vi "create_current_variables_table.vi"(7 "Step Sizes Array":dbl[](array[numeric]), 8 "error in (no error)":errorcluster, 9 "variable values":dbl[](array[numeric]), 10 "variable indices":i32[](array[numeric]), 11 "Variable Names Array":string[](array[string])) -> (0 "error out":errorcluster, 3 "Variables (Indicator)":string[][](array[string]))   [LabVIEW 2011]
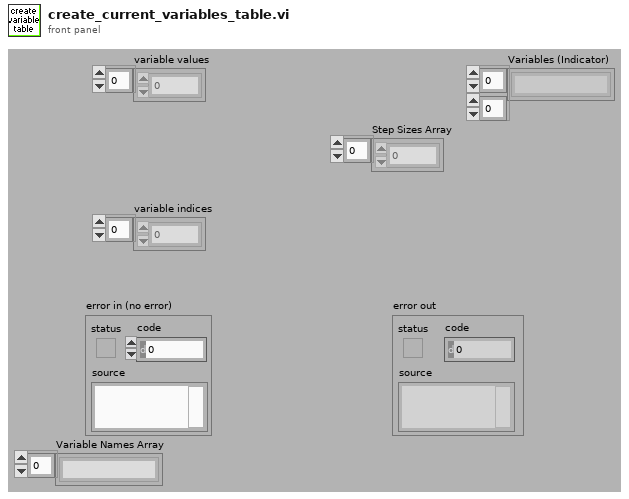
[diagram p1: front panel]
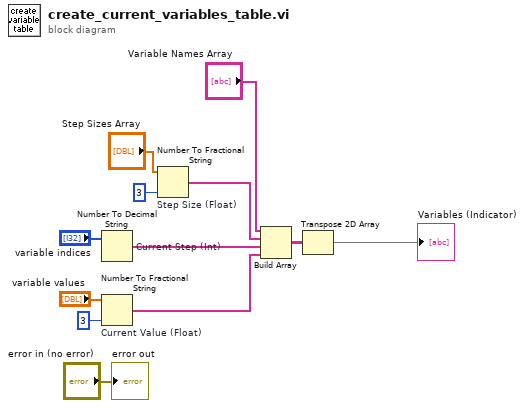
[diagram p0: block diagram]
diagram:
  n1 = Number To Decimal String "Current Step (Int)"(number="variable indices") -> (decimal integer string=w3:string[])  [unwired: 1 in]
  n2 = Number To Fractional String "Current Value (Float)"(number="variable values", precision (6)=i16 3) -> (F-format string=w2:string[])  [unwired: 2 in]
  n3 = Number To Fractional String "Step Size (Float)"(number="Step Sizes Array", precision (6)=i16 3) -> (F-format string=w4:string[])  [unwired: 2 in]
  n4 = Build Array("Variable Names Array", w4, w3, w2) -> (w1:string[][])
  n5 = Transpose 2D Array(2D array=w1) -> (transposed array=→"Variables (Indicator)":string[][])
  "error out" <- "error in (no error)"
